vi "Insert proc_Temp.vi"(8 "에러 입력(에러 없음)":errorcluster, 10 "Proc 입력":string[][](array[string])) -> (0 "에러 출력":errorcluster)   [LabVIEW 2020]
uses:
  Support/Controls/Cmd_Read Query.ctl
  Support/Controls/Clst_Query Info.ctl
  Support/Controls/Cmd_Write Query.ctl
  Variables/Global_Cal Info.vi
  <vilib>/addons/database/NI_Database_API.lvlib
  <vilib>/addons/database/Connection.llb/Conn Transaction.vi
  <vilib>/addons/database/Auxilliary.llb/DB Tools Transaction.ctl
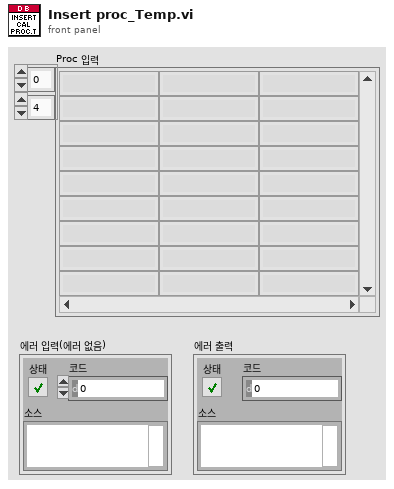
[diagram p1: front panel]
types:
  T1 = typedef "Clst_Query Info.ctl" = cluster{"사번":string, "등록번호":string, "업체명":string, "세부분류코드":string, "형식":string, "기기번호":string, "FUNC":string, "FUNC_EXT":string, "옵션":string, "추가문자열":string, "일자":string, "배열 1":string[], "배열 2":string[], "항목명":string, "문자열":string, "이름":string}
  T2 = typedef "Cmd_Read Query.ctl" = enum16{"교정자 이름 얻기", "인증교정자 얻기", "기술책임자 얻기", "기책부책 얻기", "등록번호 얻기", "등록정보 얻기", "업체정보 얻기", "교정일자(CAMAS) 얻기", "교정일자(CALSTD) 얻기", "교정환경 얻기", "교정절차서 목록 얻기", "교정절차서명 얻기", "교정절차 목록얻기", "교정절차 얻기", "PROC 교정절차 얻기", "PROC SPEC 얻기", "교정절차(Func별) 얻기", "교정절차(Func_ext별) 얻기", "기관코드 얻기", "교정기능(세부분류) 얻기", "교정기능(모델) 얻기", "교정기능 목록 얻기", "교정기능 명칭 얻기", "교정기능 항목명칭 얻기", "DB (사용기준기) 얻기", "DB (기준기이름) 얻기", "DB (기준기이름목록) 얻기", "DB (기준기목록) 얻기", "DB (기준기값) 얻기", "DB (CMC) 얻기", "DB (FUNC) 얻기", "DB (CALNAME) 얻기", "DB (STDNAME) 얻기", "DB (SPEC) 얻기", "모델(항목전체) 얻기", "모델(최대범위) 얻기", "모델(최소범위) 얻기", "모델(최대최소) 얻기", "모델(범위조건) 얻기", "모델(등록요청) 얻기", "모델(형식별) 얻기", "모델(조건별) 얻기", "모델(모델검색) 얻기", "세부분류 목록 얻기", "기준기등록리스트 얻기", "STD Cal Date Check", "DB등록일자 얻기", "적용항목 얻기", "기타정보 얻기", "기준기요청 얻기", "서버버전 얻기"}
  T3 = typedef "NI_Database_API.lvlib/Conn ObjectReference.ctl" = refnum<k1>
  T4 = typedef "Cmd_Write Query.ctl" = enum16{"TBUSESTD_MCT Insert", "TBUSESTD_MCT Delete", "TBCALSTD_MCT_TEMP Insert", "TBCALSTD_MCT_TEMP Delete", "TBCALSTD_MCT Insert", "TBCALSTD_MCT Delete", "TBCALSTD_MCT_BACK Insert", "TBCALSTD_MCT_BACK Delete", "TBCALPROC_MCT Insert", "TBCALPROC_MCT Delete", "TBCALPROC_MCT_TEMP Insert", "TBCALPROC_MCT_TEMP Delete", "TBCALCMC_MCT Insert", "TBCALCMC_MCT Delete", "TBCALFUNC_MCT Insert", "TBCALFUNC_MCT Delete", "TBCALNAME_MCT Insert", "TBCALNAME_MCT Delete", "TBSTDNAME_MCT Insert", "TBSTDNAME_MCT Delete", "TBCALSPEC_MCT Insert", "TBCALSPEC_MCT Delete", "TBCALSTD_MCT NOTUSE update", "TBCALSPEC_MCT update", "TBMCTVERMAN update"}
  T5 = typedef "NI_Database_API.lvlib/DB Tools Transaction.ctl" = enum16{"begin", "commit", "rollback"}
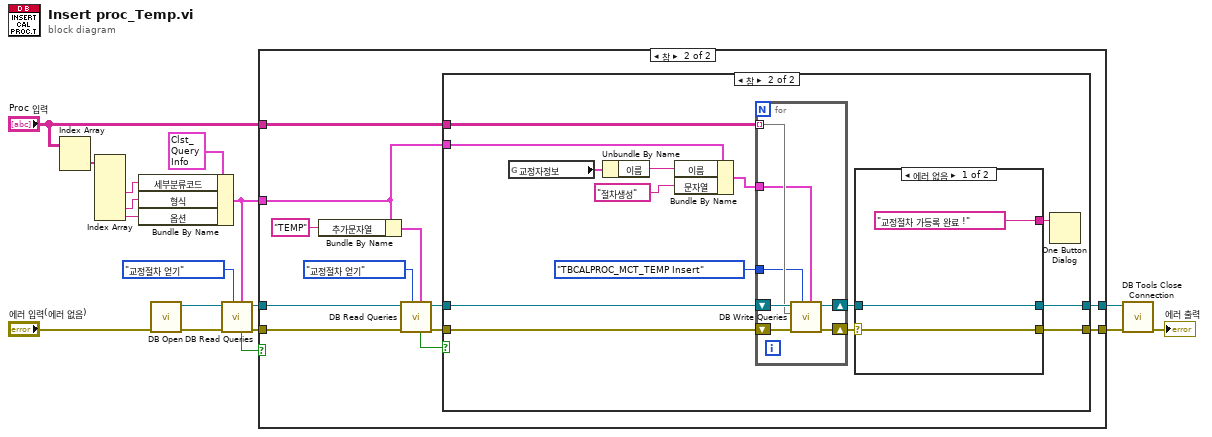
[diagram p0: block diagram]
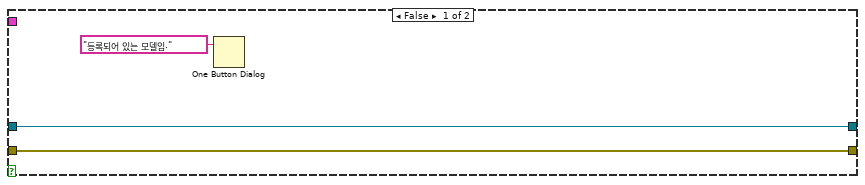
[diagram p2: hidden frame]
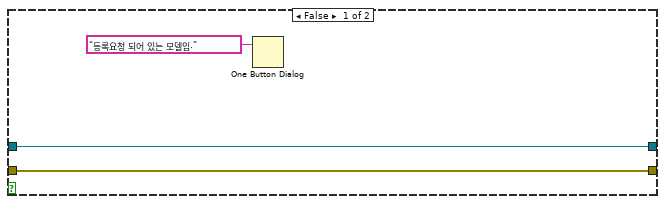
[diagram p3: hidden frame]
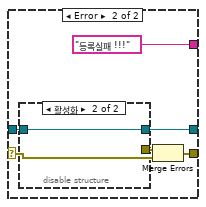
[diagram p4: hidden frame]
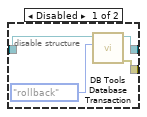
[diagram p5: hidden frame]
diagram:
  n1 = Index Array(array="Proc 입력") -> (element=w7:string[])  [unwired: 2 in]
  n2 = Index Array(array=w7) -> (element #3=w6:string, element #5=w5:string, element #6=w4:string)  [unwired: 6 in, 3 out]
  n3 = Bundle By Name(cluster=T1 {"사번"="", "등록번호"="", "업체명"="", "세부분류코드"="", "형식"="", "기기번호"="", "FUNC"="", "FUNC_EXT"="", "옵션"="", "추가문자열"="", "일자"="", "배열 1"=[], "배열 2"=[], "항목명"="", "문자열"="", "이름"=""} ("Query info"), "세부분류코드"=w6, "형식"=w5, "옵션"=w4) -> (w3:T1)
  n4 = call "DB Open.vi"("에러 입력"="에러 입력(에러 없음)") -> ("에러 출력"=w11:errorcluster, "참조 번호 출력"=w13:T3)  [unwired: 9 in]
  n5 = call "DB Read Queries.vi"("Query info"=w3, "Query Command"=Cmd_Read_Query."교정절차 얻기", "에러 입력(에러 없음)"=w11, "참조 번호 입력"=w13) -> ("에러 출력"=w12:errorcluster, "참조 번호 출력"=w14:T3, "None?"=w1:bool)  [unwired: 3 in, 2 out]
  n6 = case shown="참" w1 {
    tunnel: w14 -> [w20 w29]
    tunnel: w12 -> [w19 w30]
    tunnel: [w20 w32] -> w10
    tunnel: [w19 w31] -> w8
    tunnel: w3 -> [_ w21]
    tunnel: "Proc 입력" -> [_ w26]
    frame False {
      n7 = One Button Dialog(message="등록되어 있는 모델임." ("메시지")) -> ()  [unwired: 1 in, 1 out]
    }
    frame True {
      n8 = Bundle By Name(cluster=w21, "추가문자열"="TEMP") -> (w23:T1)
      n9 = call "DB Read Queries.vi"("Query info"=w23, "Query Command"=Cmd_Read_Query."교정절차 얻기", "에러 입력(에러 없음)"=w30, "참조 번호 입력"=w29) -> ("에러 출력"=w24:errorcluster, "참조 번호 출력"=w28:T3, "None?"=w25:bool)  [unwired: 3 in, 2 out]
      n10 = case shown="참" w25 {
        tunnel: [w34 w49] -> w32
        tunnel: [w33 w48] -> w31
        tunnel: w24 -> [w33 w45]
        tunnel: w28 -> [w34 w46]
        tunnel: w26 -> [_ w43]
        tunnel: w21 -> [_ w41]
        frame False {
          n11 = One Button Dialog(message="등록요청 되어 있는 모델임." ("메시지")) -> ()  [unwired: 1 in, 1 out]
        }
        frame True {
          n12 = global read "Global_Cal Info.vi" "교정자정보"() -> (w39:cluster{"사번":string, "이름":string, "자격":string})
          n13 = Unbundle By Name(w39) -> ("이름"=w38:string)
          n14 = Bundle By Name(cluster=w41, "이름"=w38, "문자열"="절차생성" ("항목명")) -> (w40:T1)
          n15 = for {
            tunnel: w43 -> [w52] mode=indexing
            shift-right: [w56] -> w47
            shift-left: w46 -> [w55]
            shift-right: [w53] -> w44
            shift-left: w45 -> [w54]
            tunnel: w40 -> [w51]
            tunnel: Cmd_Write_Query."TBCALPROC_MCT_TEMP Insert" ("COMMAND") -> [w50]
            n16 = call "DB Write Queries.vi"("Query info"=w51, "COMMAND"=w50, "에러 입력(에러 없음)"=w54, "DATA IN"=w52, "참조 번호 입력"=w55) -> ("에러 출력"=w53:errorcluster, "참조 번호 출력"=w56:T3)  [unwired: 5 in]
          }
          n17 = case shown="에러 없음" w44 {
            selector: w44 -> [w58 w63]
            tunnel: [w59 w65] -> w49
            tunnel: w47 -> [w59 w64]
            tunnel: [w58 w62] -> w48
            tunnel: ["교정절차 가등록 완료 !" "등록실패 !!!"] -> w42
            frame No Error {
            }
            frame Error {
              n18 = disable-structure shown="활성화" {
                disable-tunnel: [w69 w70] -> w65
                disable-tunnel: w64 -> [w68 w70]
                disable-tunnel: [w66 _] -> w61
                frame Disabled {
                  n19 = call-poly <vilib>:"DB Tools Database Transaction.vi"("operation (begin)"=DB_Tools_Transaction."rollback", "connection reference"=w68) -> ("error out"=w66:errorcluster, "connection reference out"=w69:T3)  [unwired: 4 in]
                }
                frame Enabled {
                }
              }
              n20 = Merge Errors(w61, w63) -> (w62:errorcluster)
            }
          }
          n21 = One Button Dialog(message=w42) -> ()  [unwired: 1 in, 1 out]
        }
      }
    }
  }
  n22 = call <vilib>:"DB Tools Close Connection.vi"("error in (no error)"=w8, "connection reference"=w10) -> ("error out"=→"에러 출력":errorcluster)  [unwired: 5 in]
